vi "ROS_Register.vi"(2 "Parameters":string[](array[string]), 3 "Method Name":string) -> (1 "registerSubscriber":string="POST /RPC2 HTTP/1.1\r\nHost: 192.168.1.110:11311\r\nContent-Type: text/xml\r\nContent-Length: 396\r\n\r\n<?xml version='1.0'?>\n<methodCall>\r <methodName>registerSubscriber</methodName>\r <params>\r   <param><value><string>/ChrisAir</string> </value> </param>\r   <param><value><string>/robot/joint_states</string> </value> </param>\r   <param><value><string>sensor_msgs/JointState</string> </value> </param>\r   <param><value><string>http://192.168.1.111</string> </value> </param>\r </params>\r</methodCall>")   [LabVIEW 2012]
doc: "Registers and unregisters topics"
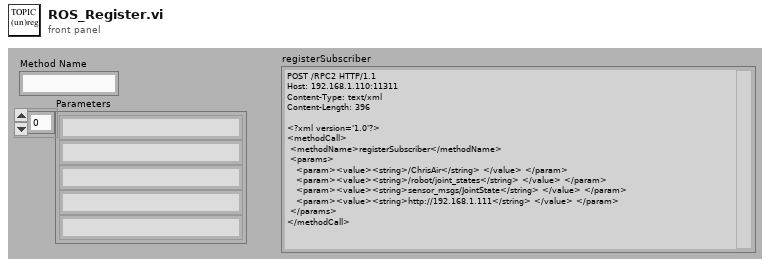
[diagram p1: front panel]
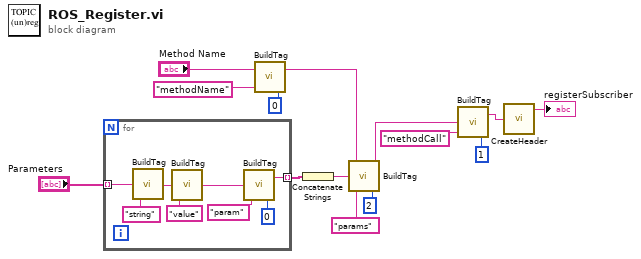
[diagram p0: block diagram]
diagram:
  n1 = for {
    tunnel: "Parameters" -> [w16] mode=indexing
    tunnel: [w15] -> w12 mode=indexing
    n2 = call "BuildTag.vi"("tag"="string", "value"=w16) -> ("string out"=w20:string)  [unwired: 2 in]
    n3 = call "BuildTag.vi"("tag"="value", "value"=w20) -> ("string out"=w18:string)  [unwired: 2 in]
    n4 = call "BuildTag.vi"("Indent"=i8 0, "tag"="param", "value"=w18) -> ("string out"=w15:string)  [unwired: 1 in]
  }
  n5 = call "BuildTag.vi"("Indent"=i8 0, "tag"="methodName", "value"="Method Name") -> ("string out"=w7:string)  [unwired: 1 in]
  n6 = Concatenate Strings(w12) -> (w13:string)
  n7 = call "BuildTag.vi"("Indent"=i8 2, "tag"="params", "value"=w13, "string in"=w7) -> ("string out"=w4:string)
  n8 = call "BuildTag.vi"("Indent"=i8 1, "tag"="methodCall", "value"=w4) -> ("string out"=w10:string)  [unwired: 1 in]
  n9 = call "CreateHeader.vi"("Content"=w10) -> ("XML"=→"registerSubscriber":string)
